vi "queue2.vi"() -> ()   [LabVIEW 2018]
panel:
  in  "Texto":string
  in  "?":bool
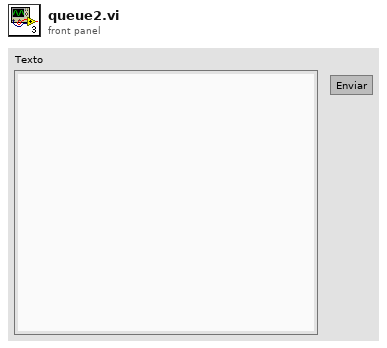
[diagram p1: front panel]
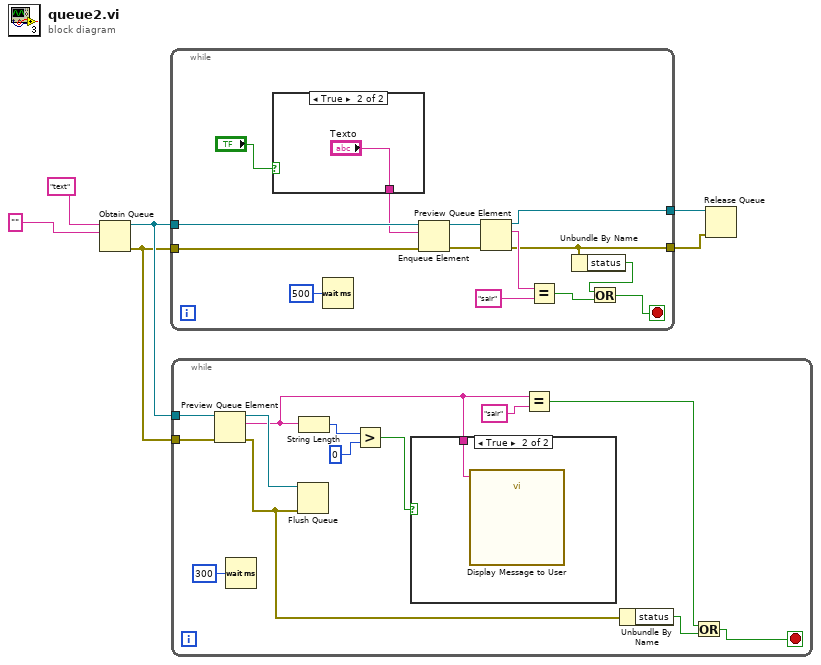
[diagram p0: block diagram]
diagram:
  n1 = Obtain Queue(name (unnamed)="text", element data type="") -> (queue out=w2:refnum<queue>, error out=w1:errorcluster)  [unwired: 3 in, 1 out]
  n2 = while {
    tunnel: w2 -> [w19]
    tunnel: w1 -> [w18]
    tunnel: [w12] -> w4
    tunnel: [w11] -> w3
    stop <- w8 stop-if-true
    n3 = case shown="True" "?" {
      tunnel: [_ "Texto"] -> w17
      frame False {
      }
      frame True {
      }
    }
    n4 = Wait (ms)(milliseconds to wait=u32 500) -> ()  [unwired: 1 out]
    n5 = Enqueue Element(queue=w19, element=w17, error in (no error)=w18) -> (queue out=w15:refnum<queue>, error out=w16:errorcluster)  [unwired: 1 in, 1 out]
    n6 = Preview Queue Element(queue=w15, error in (no error)=w16) -> (queue out=w12:refnum<queue>, element=w14:string, error out=w11:errorcluster)  [unwired: 1 in, 1 out]
    n7 = Equal?(x=w14, y="sair") -> (x = y?=w9:bool)
    n8 = Unbundle By Name(w11) -> ("status"=w10:bool)
    n9 = Or(x=w10, y=w9) -> (x .or. y?=w8:bool)
  }
  n10 = while {
    tunnel: w2 -> [w34]
    tunnel: w1 -> [w33]
    stop <- w22 stop-if-true
    n11 = Preview Queue Element(queue=w34, error in (no error)=w33) -> (queue out=w29:refnum<queue>, element=w27:string, error out=w25:errorcluster)  [unwired: 1 in, 1 out]
    n12 = Wait (ms)(milliseconds to wait=u32 300) -> ()  [unwired: 1 out]
    n13 = Flush Queue(queue=w29, error in (no error)=w25) -> ()  [unwired: 3 out]
    n14 = String Length(string=w27) -> (length=w32:i32)
    n15 = Greater?(x=w32, y=0) -> (0:w30:bool)
    n16 = case shown="True" w30 {
      tunnel: w27 -> [_ w35]
      frame False {
      }
      frame True {
        n17 = call "Display Message to User"("Message"=w35) -> ()  [unwired: 9 in, 2 out]
      }
    }
    n18 = Equal?(x=w27, y="sair") -> (x = y?=w24:bool)
    n19 = Unbundle By Name(w25) -> ("status"=w23:bool)
    n20 = Or(x=w24, y=w23) -> (x .or. y?=w22:bool)
  }
  n21 = Release Queue(queue=w4, error in (no error)=w3) -> ()  [unwired: 1 in, 3 out]
